vi "Halvorsen_Effect_Graph.vi"() -> ()   [LabVIEW 2016]
panel:
  in  "Parameters array":dbl[](array[numeric])=[1.4, 1.4, 1.4]
  in  "last_point_Thomas":dbl[](array[numeric])=[2.3727475682665875, 0.23609824454436878, 0.4447912442126299]
  out "Efficiency plot":cluster{dbl[], dbl[]}[](graph)=[{[0.003543503530615683, 0.008857469273654535, 0.00019032089210001206, 1.3154265970568985e-05, 7.569954419870983e-07, 2.611584956422264e-08, 5.111791074846327e-10, 1.2810097409899129e-09, 1.4983661356938417e-09, 8.704238501746543e-11], [0.0006568757962668315, 0.0006969041642150842, 0.001332226223894395, 0.0013178570661693811, 0.001516972541139694, 0.0019039134404010838, 0.002382201128966699, 0.0033203018756466918, 0.004479071834794013, 0.006073022008422413]}, {[0.05292939277385792, 0.005366821516305654, 0.00032764804221647705, 2.8472873719995087e-05, 1.7555059222208518e-06, 2.2173371174251578e-07, 4.046899467880833e-09, 2.1493117845000048e-09, 1.62941200420686e-09, 7.302730760301067e-09], [0.0007903036921561579, 0.0010448430630276562, 0.001373280961161072, 0.0016955606479314156, 0.003905331881469465, 0.0027578519757298636, 0.004559128571600013, 0.00517905510514538, 0.007503779601393035, 0.010119992733962135]}, {[0.002038488022454064, 0.000645465458210278, 0.00017338121373700052, 3.264021324537677e-05, 2.183623841080202e-06, 1.9365539284403195e-07, 2.508911679074605e-08, 3.0422395440576762e-09, 1.1221599069650436e-10, 1.6048322905065433e-09], [0.0009863400628091767, 0.0013722545927521423, 0.0017335362808807986, 0.0021943757055851165, 0.0030134177141007967, 0.0041157374098474975, 0.005651184582347923, 0.007658761235688871, 0.010887716319302854, 0.015299047837288526]}, {[0.0065546151240054125, 0.003030290222989306, 0.0008963869972767443, 8.930764045777448e-05, 2.652903337131928e-05, 1.0284405279190207e-06, 9.203396690137426e-08, 1.058326598406588e-08, 1.8330857120193038e-09, 8.540691445443122e-11], [0.0007246161130751716, 0.0009391271141794277, 0.0012429321695890394, 0.0016863233322510496, 0.0021256090221868362, 0.0027855639227709617, 0.0037452184060384752, 0.004844458995648893, 0.006607759961298143, 0.00915212730251369]}, {[0.031777470957385985, 0.0021554762412673728, 9.17895270926683e-05, 1.7052624686084191e-06, 6.452919290133345e-07, 4.7099078030656e-08, 8.99697945269555e-09, 4.212593948523254e-10, 1.4960189944277468e-10, 8.913127927436747e-10], [0.000523447900377505, 0.0006219792694537318, 0.0008467539555567782, 0.0011053988009734894, 0.0014461531200140598, 0.001842331334046321, 0.002354489181925601, 0.0033921476651812554, 0.0042563498855088255, 0.00598783342866227]}, {[0.01953779155905403, 0.011210076118577949, 0.0003345025752221787, 1.698158066222403e-06, 1.2746234512715955e-06, 2.029307378175867e-08, 3.577829362814558e-10, 3.945270287029524e-10, 2.68884023315538e-10, 2.253025074843069e-09], [0.000610689216046012, 0.0007636181126144947, 0.0014882342256896663, 0.0017171143863379257, 0.0023165135498857126, 0.0021687164962713723, 0.0025628419725762797, 0.0038991736710158875, 0.005071286419479293, 0.006304981274297461]}, {[0.644522862841223, 0.07384111446896484, 0.038699076952541156, 0.00422549784591777, 0.0006539084545961815, 0.0001447132168707633, 3.4362296547381575e-05, 6.549119527339312e-06, 6.89087435666376e-06, 1.0243970291599666e-05], [0.0008467539555567782, 0.0011567172214199672, 0.0017591954920135322, 0.0029518356086555286, 0.004991229681763798, 0.008791871982793964, 0.015572061841339746, 0.0268436399546772, 0.045662105143492226, 0.06235393494262098]}, {[0.06903372684326185, 0.00020304900818616015, 8.637150762520324e-05, 1.689029168945209e-06, 8.057455570285068e-07, 2.9659954301410987e-08, 2.4135215284240776e-09, 1.1473823618093083e-09, 6.606131463009407e-10, 6.428058997780049e-10], [0.0005727135840061237, 0.0006989569010329433, 0.0009688917998573743, 0.0012860396445830702, 0.0016996661224766285, 0.003623080562647374, 0.002643925078700704, 0.00331311729587469, 0.0048054569961095694, 0.006534887802445155]}, {[0.009934991568151866, 0.001930410234965607, 5.014437765295048e-05, 1.7981970136881245e-05, 5.418162911083816e-06, 1.00173853871348e-06, 2.4670319318787825e-07, 3.898500256142404e-08, 5.109251324047994e-09, 3.051511094268924e-10], [0.005962174217529537, 0.008118574292893754, 0.009580122939041757, 0.012024932541862654, 0.01608421968830953, 0.021048763790531666, 0.02561712967872154, 0.03248045537930011, 0.04417387091780256, 0.06094370471782895]}]
  in  "Multipliers":i32[](array[numeric])=[2, 2, 2, 2, 2, 2, 2, 2, 2, 2, 2, 2, 2]
  in  "Methods":u16[](array[ring])=[0, 4, 5, 9, 1, 2, 6, 3, 10] items=["ECD1", "ECD2", "ECD3", "ECD4", "EMP", "LIMP", "SEMP", "SIMP", "Euler", "MEMP", "IMP", "IEuler", "MSEMP"]
  in  "Tab Control":enum32{"Variable step", "Fixed Step"}(tab)
  in  "Tolerances":dbl[](array[numeric])=[0.0001, 1e-05, 1e-06, 1e-07, 1e-08, 1e-09, 1e-10, 1e-11, 1e-12, 1e-13]
  in  "Max Steps":dbl[](array[numeric])=[2.0, 2.0, 2.0, 2.0, 2.0, 2.0, 2.0, 2.0, 2.0, 2.0]
  in  "Start steps":dbl[](array[numeric])=[0.01, 0.01, 0.01, 0.01, 0.01, 0.01, 0.01, 0.01, 0.01, 0.04]
  in  "Min Steps":dbl[](array[numeric])=[0.001, 0.001, 0.001, 0.001, 0.001, 0.001, 0.001, 0.001, 0.001, 0.001]
  in  "Tolerances 2":dbl[](array[numeric])=[1e-06, 1e-06, 1e-06, 1e-06, 1e-06, 1e-06, 1e-06, 1e-06, 1e-06]
  in  "Start steps 2":dbl[](array[numeric])=[2.0, 1.0, 0.4, 0.3, 0.2, 0.1, 0.08, 0.05, 0.02, 0.01]
  out "Rejected":i32[][](array[numeric])=[[11, 16, 10, 11, 8, 11, 14, 10, 11], [12, 18, 13, 14, 9, 9, 15, 12, 12], [14, 24, 13, 18, 13, 16, 14, 16, 15], [16, 19, 17, 22, 16, 16, 17, 19, 16], [16, 14, 19, 18, 16, 17, 18, 17, 21], [15, 6, 16, 12, 14, 18, 19, 19, 25], [7, 3, 9, 8, 8, 12, 20, 11, 17], [5, 2, 1, 2, 2, 5, 22, 6, 2], [5, 2, 1, 0, 0, 3, 24, 4, 2], [5, 2, 2, 1, 1, 3, 21, 3, 1]]
  in  "Points count":i32=1
  in  "Ext.Type":u16(ring) items=["FNode", "MathScript", "ECD8 Arrays", "ECD8 Fnode", "ECD8 FnodeDiv", "FNode Exp"]
  in  "?":bool
  in  "n_2":i32[](array[numeric])=[2, 3, 4, 5, 8, 10, 12, 14, 16, 10, 11]
  in  "n_1":i32[](array[numeric])=[1, 2, 3, 4, 5, 6, 7, 8, 9, 10, 11]
  out "Times":dbl[][](array[numeric])=[[0.0006568757962668315, 0.0007903036921561579, 0.0009863400628091767, 0.0007246161130751716, 0.000523447900377505, 0.000610689216046012, 0.0008467539555567782, 0.0005727135840061237, 0.005962174217529537], [0.0006969041642150842, 0.0010448430630276562, 0.0013722545927521423, 0.0009391271141794277, 0.0006219792694537318, 0.0007636181126144947, 0.0011567172214199672, 0.0006989569010329433, 0.008118574292893754], [0.001332226223894395, 0.001373280961161072, 0.0017335362808807986, 0.0012429321695890394, 0.0008467539555567782, 0.0014882342256896663, 0.0017591954920135322, 0.0009688917998573743, 0.009580122939041757], [0.0013178570661693811, 0.0016955606479314156, 0.0021943757055851165, 0.0016863233322510496, 0.0011053988009734894, 0.0017171143863379257, 0.0029518356086555286, 0.0012860396445830702, 0.012024932541862654], [0.001516972541139694, 0.003905331881469465, 0.0030134177141007967, 0.0021256090221868362, 0.0014461531200140598, 0.0023165135498857126, 0.004991229681763798, 0.0016996661224766285, 0.01608421968830953], [0.0019039134404010838, 0.0027578519757298636, 0.0041157374098474975, 0.0027855639227709617, 0.001842331334046321, 0.0021687164962713723, 0.008791871982793964, 0.003623080562647374, 0.021048763790531666], [0.002382201128966699, 0.004559128571600013, 0.005651184582347923, 0.0037452184060384752, 0.002354489181925601, 0.0025628419725762797, 0.015572061841339746, 0.002643925078700704, 0.02561712967872154], [0.0033203018756466918, 0.00517905510514538, 0.007658761235688871, 0.004844458995648893, 0.0033921476651812554, 0.0038991736710158875, 0.0268436399546772, 0.00331311729587469, 0.03248045537930011], [0.004479071834794013, 0.007503779601393035, 0.010887716319302854, 0.006607759961298143, 0.0042563498855088255, 0.005071286419479293, 0.045662105143492226, 0.0048054569961095694, 0.04417387091780256], [0.006073022008422413, 0.010119992733962135, 0.015299047837288526, 0.00915212730251369, 0.00598783342866227, 0.006304981274297461, 0.06235393494262098, 0.006534887802445155, 0.06094370471782895]] format="%#_10f"
  out "Steps":i32[][](array[numeric])=[[28, 50, 28, 43, 27, 27, 55, 27, 27], [34, 66, 37, 58, 34, 33, 79, 34, 35], [45, 91, 49, 77, 46, 45, 130, 46, 45], [61, 120, 65, 104, 62, 61, 225, 66, 59], [83, 164, 89, 140, 84, 83, 396, 86, 80], [115, 225, 121, 191, 114, 116, 702, 117, 108], [156, 311, 166, 263, 156, 156, 1249, 159, 146], [216, 431, 229, 364, 215, 215, 2200, 220, 200], [299, 599, 320, 505, 298, 298, 3548, 305, 278], [415, 831, 444, 701, 414, 413, 4777, 424, 386]]
  out "Errors":dbl[][](array[numeric])=[[0.003543503530615683, 0.05292939277385792, 0.002038488022454064, 0.0065546151240054125, 0.031777470957385985, 0.01953779155905403, 0.644522862841223, 0.06903372684326185, 0.009934991568151866], [0.008857469273654535, 0.005366821516305654, 0.000645465458210278, 0.003030290222989306, 0.0021554762412673728, 0.011210076118577949, 0.07384111446896484, 0.00020304900818616015, 0.001930410234965607], [0.00019032089210001206, 0.00032764804221647705, 0.00017338121373700052, 0.0008963869972767443, 9.17895270926683e-05, 0.0003345025752221787, 0.038699076952541156, 8.637150762520324e-05, 5.014437765295048e-05], [1.3154265970568985e-05, 2.8472873719995087e-05, 3.264021324537677e-05, 8.930764045777448e-05, 1.7052624686084191e-06, 1.698158066222403e-06, 0.00422549784591777, 1.689029168945209e-06, 1.7981970136881245e-05], [7.569954419870983e-07, 1.7555059222208518e-06, 2.183623841080202e-06, 2.652903337131928e-05, 6.452919290133345e-07, 1.2746234512715955e-06, 0.0006539084545961815, 8.057455570285068e-07, 5.418162911083816e-06], [2.611584956422264e-08, 2.2173371174251578e-07, 1.9365539284403195e-07, 1.0284405279190207e-06, 4.7099078030656e-08, 2.029307378175867e-08, 0.0001447132168707633, 2.9659954301410987e-08, 1.00173853871348e-06], [5.111791074846327e-10, 4.046899467880833e-09, 2.508911679074605e-08, 9.203396690137426e-08, 8.99697945269555e-09, 3.577829362814558e-10, 3.4362296547381575e-05, 2.4135215284240776e-09, 2.4670319318787825e-07], [1.2810097409899129e-09, 2.1493117845000048e-09, 3.0422395440576762e-09, 1.058326598406588e-08, 4.212593948523254e-10, 3.945270287029524e-10, 6.549119527339312e-06, 1.1473823618093083e-09, 3.898500256142404e-08], [1.4983661356938417e-09, 1.62941200420686e-09, 1.1221599069650436e-10, 1.8330857120193038e-09, 1.4960189944277468e-10, 2.68884023315538e-10, 6.89087435666376e-06, 6.606131463009407e-10, 5.109251324047994e-09], [8.704238501746543e-11, 7.302730760301067e-09, 1.6048322905065433e-09, 8.540691445443122e-11, 8.913127927436747e-10, 2.253025074843069e-09, 1.0243970291599666e-05, 6.428058997780049e-10, 3.051511094268924e-10]] format="%#_9e"
  in  "Время, с":dbl=5.0
  in  "k":i32=4
  in  "Error Analysis":u16(ring)=2 items=["Max", "Max_Norm", "Norm", "Last Value", "Last Constant"]
  # "0 ECD1\n1 ECD2\n2 ECD3\n3 ECD4\n4 EMP\n5 LIMP\n6 SEMP\n7 SIMP\n8 Euler\n9 Euler-Cromer\n10 MECD1\n11 MECD2\n12 MECD3\n13 MECD4\n14 MEMP\n15 MLIMP\n16 MSEMP\n17 MSIMP"
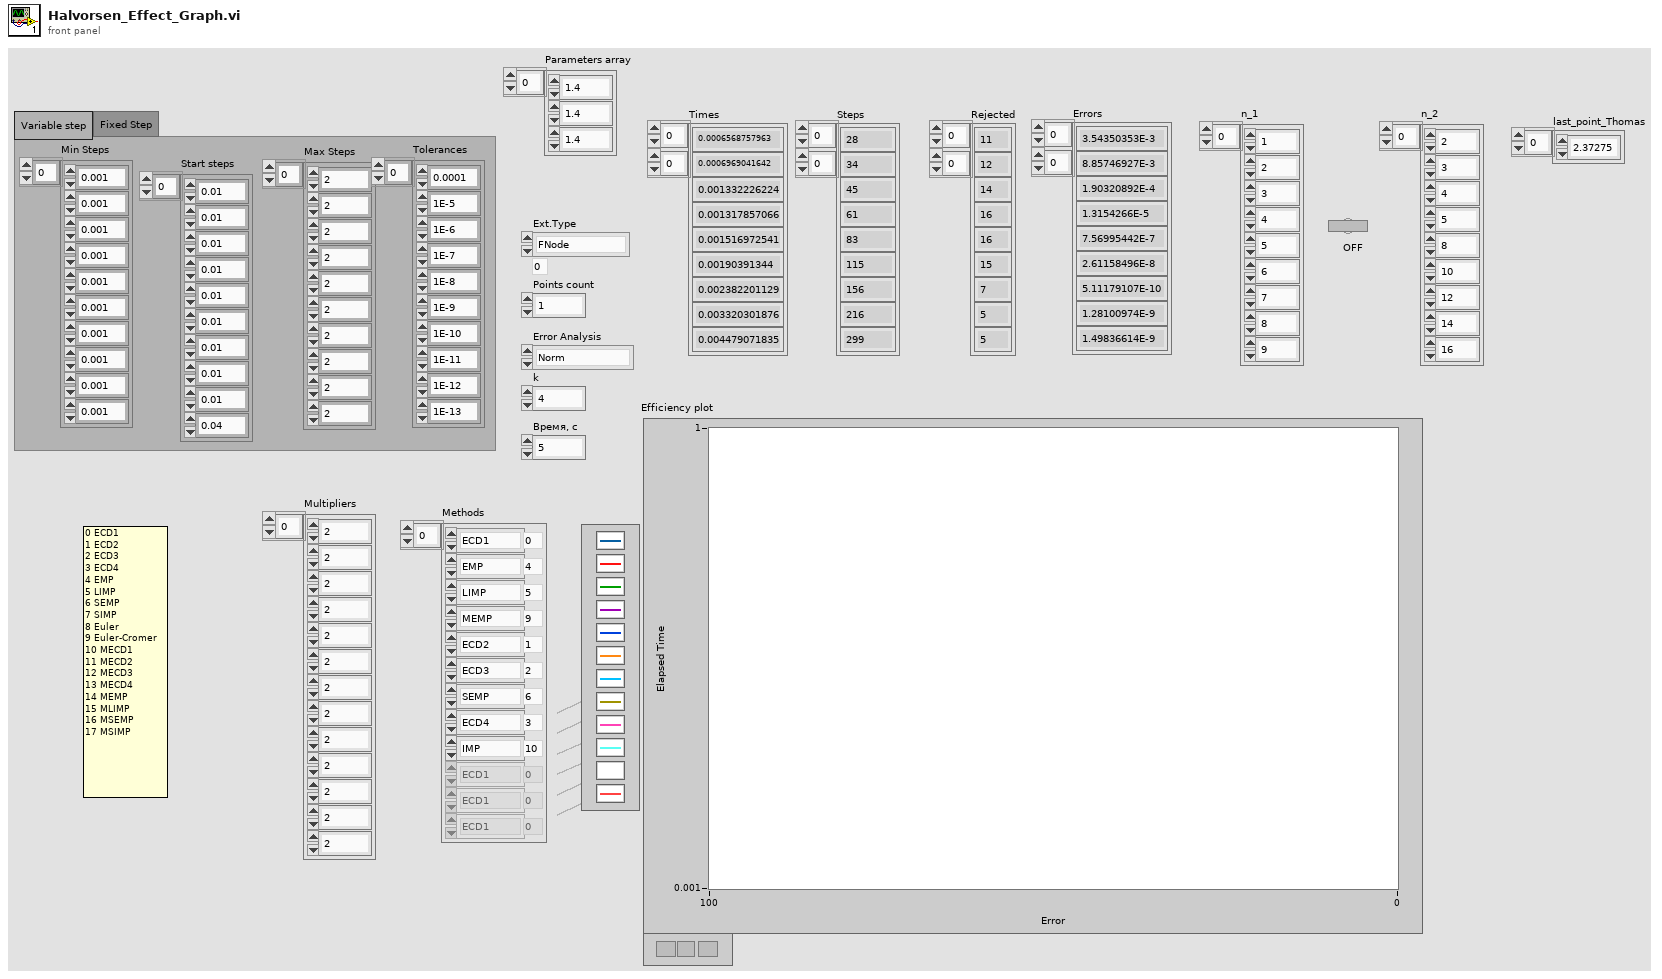
[diagram p1: front panel]
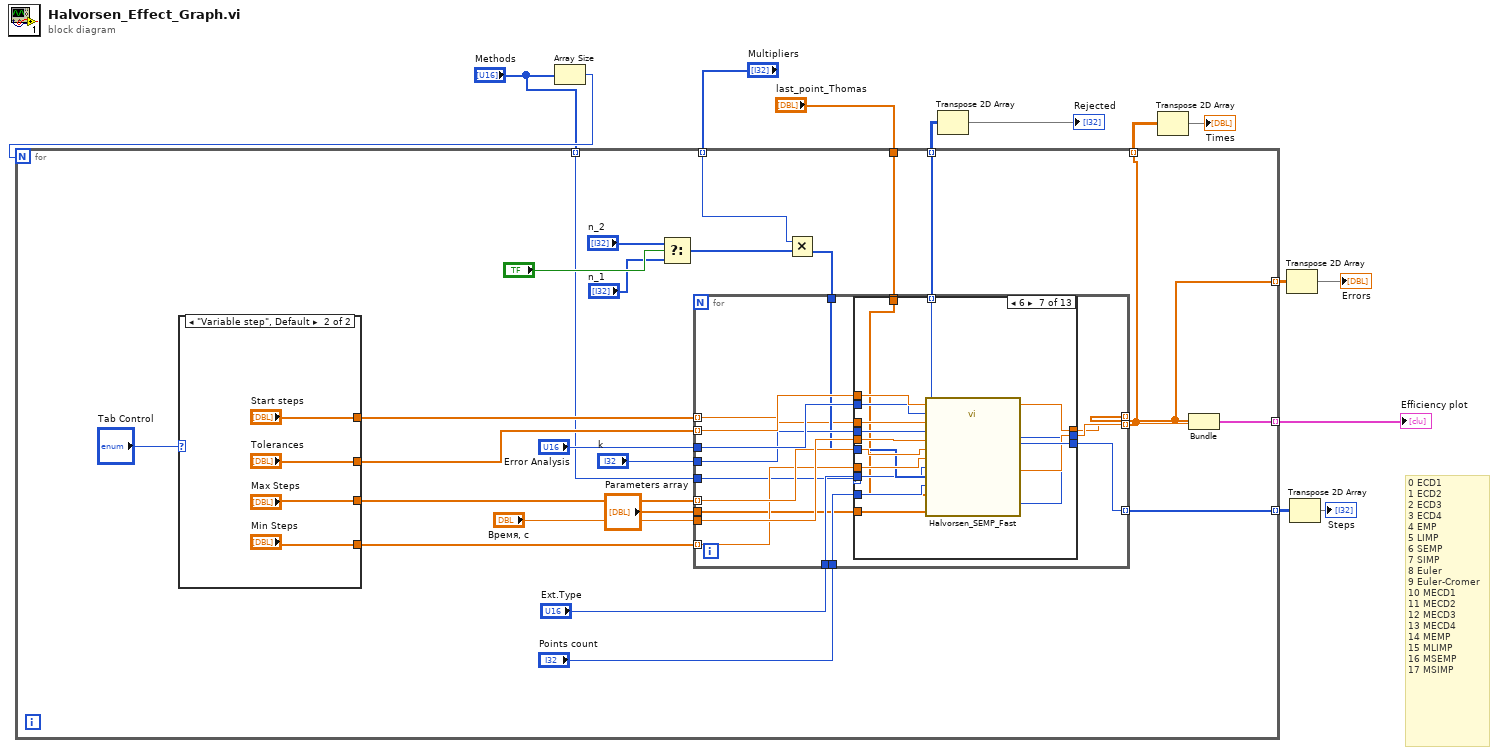
[diagram p0: block diagram]
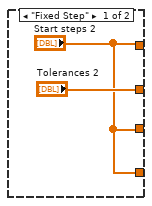
[diagram p2: hidden frame]
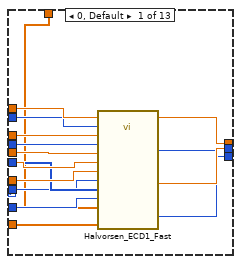
[diagram p3: hidden frame]
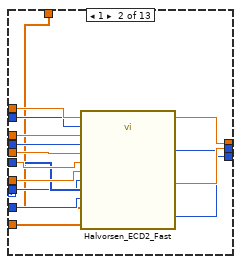
[diagram p4: hidden frame]
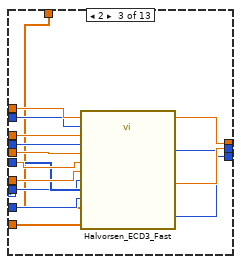
[diagram p5: hidden frame]
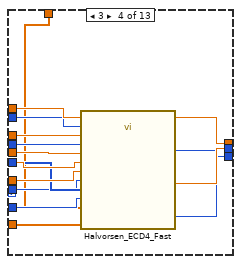
[diagram p6: hidden frame]
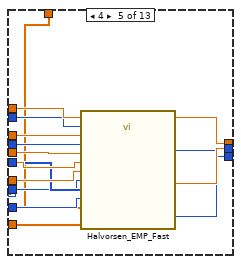
[diagram p7: hidden frame]
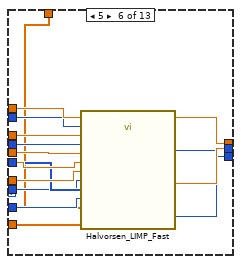
[diagram p8: hidden frame]
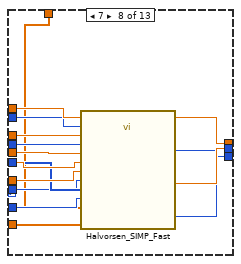
[diagram p9: hidden frame]
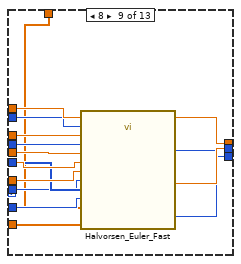
[diagram p10: hidden frame]
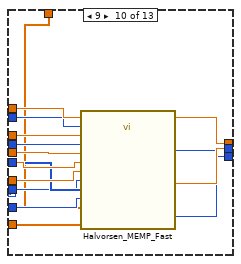
[diagram p11: hidden frame]
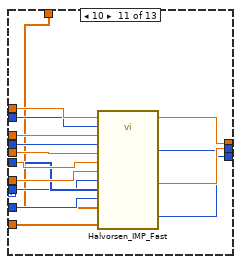
[diagram p12: hidden frame]
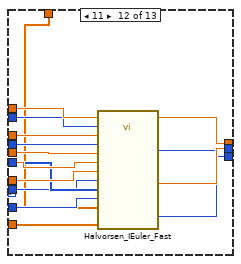
[diagram p13: hidden frame]
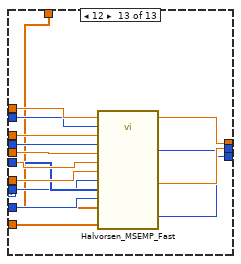
[diagram p14: hidden frame]
diagram:
  # "0 ECD1\n1 ECD2\n2 ECD3\n3 ECD4\n4 EMP\n5 LIMP\n6 SEMP\n7 SIMP\n8 Euler\n9 Euler-Cromer\n10 MECD1\n11 MECD2\n12 MECD3\n13 MECD4\n14 MEMP\n15 MLIMP\n16 MSEMP\n17 MSIMP"
  n1 = Array Size(array="Methods") -> (size(s)=w5:i32)
  n2 = for {
    N: w5 -> [_]
    tunnel: [w22] -> w2 mode=indexing
    tunnel: [w21] -> w13 mode=indexing
    tunnel: [w20] -> w12 mode=indexing
    tunnel: [w19] -> w11 mode=indexing
    tunnel: [w18] -> w10 mode=indexing
    tunnel: "Methods" -> [w17] mode=indexing
    tunnel: "Multipliers" -> [w16] mode=indexing
    tunnel: "last_point_Thomas" -> [w15]
    n3 = case shown="\"Variable step\", Default" "Tab Control" {
      tunnel: ["Tolerances 2" "Tolerances"] -> w37
      tunnel: ["Start steps 2" "Start steps"] -> w26
      tunnel: ["Start steps 2" "Max Steps"] -> w25
      tunnel: ["Start steps 2" "Min Steps"] -> w24
      frame "Fixed Step" {
      }
      frame "Variable step", Default {
      }
    }
    n4 = Select(t="n_2", s="?", f="n_1") -> (s? t:f=w32:i32[])
    n5 = Multiply(x=w16, y=w32) -> (x*y=w33:i32[])
    n6 = for {
      tunnel: w37 -> [w60] mode=indexing
      tunnel: "Error Analysis" -> [w59]
      tunnel: "k" -> [w58]
      tunnel: "Время, с" -> [w57]
      tunnel: w25 -> [w56] mode=indexing
      tunnel: w24 -> [w55] mode=indexing
      tunnel: w33 -> [w54]
      tunnel: [w53] -> w18 mode=indexing
      tunnel: [w52] -> w19 mode=indexing
      tunnel: [w51] -> w21 mode=indexing
      tunnel: "Ext.Type" -> [w50]
      tunnel: "Points count" -> [w49]
      tunnel: [w48] -> w20 mode=indexing
      tunnel: w26 -> [w47] mode=indexing
      tunnel: w17 -> [w46]
      tunnel: w15 -> [w45]
      tunnel: "Parameters array" -> [w44]
      n7 = case shown="6" w46 {
        tunnel: w60 -> [w76 w92 w108 w124 w140 w156 w172 w188 w204 w220 w236 w252 w268]
        tunnel: w59 -> [w75 w91 w107 w123 w139 w155 w171 w187 w203 w219 w235 w251 w267]
        tunnel: w58 -> [w74 w90 w106 w122 w138 w154 w170 w186 w202 w218 w234 w250 w266]
        tunnel: w57 -> [w73 w89 w105 w121 w137 w153 w169 w185 w201 w217 w233 w249 w265]
        tunnel: w56 -> [w72 w88 w104 w120 w136 w152 w168 w184 w200 w216 w232 w248 w264]
        tunnel: w55 -> [w71 w87 w103 w119 w135 w151 w167 w183 w199 w215 w231 w247 w263]
        tunnel: w54 -> [w70 w86 w102 w118 w134 w150 w166 w182 w198 w214 w230 w246 w262]
        tunnel: [w69 w85 w101 w117 w133 w149 w165 w181 w197 w213 w229 w245 w261] -> w53
        tunnel: [w68 w84 w100 w116 w132 w148 w164 w180 w196 w212 w228 w244 w260] -> w52
        tunnel: [w67 w83 w99 w115 w131 w147 w163 w179 w195 w211 w227 w243 w259] -> w51
        tunnel: w50 -> [w66 w82 w98 w114 w130 w146 w162 w178 w194 w210 w226 w242 w258]
        tunnel: w49 -> [w65 w81 w97 w113 w129 w145 w161 w177 w193 w209 w225 w241 w257]
        tunnel: [w64 w80 w96 w112 w128 w144 w160 w176 w192 w208 w224 w240 w256] -> w48
        tunnel: w47 -> [w63 w79 w95 w111 w127 w143 w159 w175 w191 w207 w223 w239 w255]
        tunnel: w45 -> [w62 w78 w94 w110 w126 w142 w158 w174 w190 w206 w222 w238 w254]
        tunnel: w44 -> [w61 w77 w93 w109 w125 w141 w157 w173 w189 w205 w221 w237 w253]
        frame 0, Default {
          n8 = call "Halvorsen_ECD1_Fast.vi"("tolerance"=w76, "Error Analysis"=w75, "Шаг h, с"=w63, "k"=w74, "Время, с"=w73, "Hmax"=w72, "b"=w61, "last_point_Thomas"=w62, "Hmin"=w71, "Points count"=w65, "n"=w70, "Ext.Type"=w66) -> ("Elapsed Time"=w69:dbl, "Number of steps"=w67:i32, "Error Estimation"=w68:dbl, "Rejected steps"=w64:i32)  [unwired: 4 in]
        }
        frame 1 {
          n9 = call "Halvorsen_ECD2_Fast.vi"("tolerance"=w92, "Error Analysis"=w91, "Шаг h, с"=w79, "k"=w90, "Время, с"=w89, "Hmax"=w88, "b"=w77, "last_point_Thomas"=w78, "Hmin"=w87, "Points count"=w81, "n"=w86, "Ext.Type"=w82) -> ("Elapsed Time"=w85:dbl, "Number of steps"=w83:i32, "Error Estimation"=w84:dbl, "Rejected steps"=w80:i32)  [unwired: 4 in]
        }
        frame 2 {
          n10 = call "Halvorsen_ECD3_Fast.vi"("tolerance"=w108, "Error Analysis"=w107, "Шаг h, с"=w95, "k"=w106, "Время, с"=w105, "Hmax"=w104, "b"=w93, "last_point_Thomas"=w94, "Hmin"=w103, "Points count"=w97, "n"=w102, "Ext.Type"=w98) -> ("Elapsed Time"=w101:dbl, "Number of steps"=w99:i32, "Error Estimation"=w100:dbl, "Rejected steps"=w96:i32)  [unwired: 4 in]
        }
        frame 3 {
          n11 = call "Halvorsen_ECD4_Fast.vi"("tolerance"=w124, "Error Analysis"=w123, "Шаг h, с"=w111, "k"=w122, "Время, с"=w121, "Hmax"=w120, "b"=w109, "last_point_Thomas"=w110, "Hmin"=w119, "Points count"=w113, "n"=w118, "Ext.Type"=w114) -> ("Elapsed Time"=w117:dbl, "Number of steps"=w115:i32, "Error Estimation"=w116:dbl, "Rejected steps"=w112:i32)  [unwired: 4 in]
        }
        frame 4 {
          n12 = call "Halvorsen_EMP_Fast.vi"("tolerance"=w140, "Error Analysis"=w139, "Шаг h, с"=w127, "k"=w138, "Время, с"=w137, "Hmax"=w136, "Parameter"=w125, "last_point_Thomas"=w126, "Hmin"=w135, "Points count"=w129, "n"=w134, "Ext.Type"=w130) -> ("Elapsed Time"=w133:dbl, "Number of steps"=w131:i32, "Error Estimation"=w132:dbl, "Rejected steps"=w128:i32)  [unwired: 4 in]
        }
        frame 5 {
          n13 = call "Halvorsen_LIMP_Fast.vi"("tolerance"=w156, "Error Analysis"=w155, "Шаг h, с"=w143, "k"=w154, "Время, с"=w153, "Hmax"=w152, "Parameter"=w141, "last_point_Thomas"=w142, "Hmin"=w151, "Points count"=w145, "n"=w150, "Ext.Type"=w146) -> ("Elapsed Time"=w149:dbl, "Number of steps"=w147:i32, "Error Estimation"=w148:dbl, "Rejected steps"=w144:i32)  [unwired: 4 in]
        }
        frame 6 {
          n14 = call "Halvorsen_SEMP_Fast.vi"("tolerance"=w172, "Error Analysis"=w171, "Шаг h, с"=w159, "k"=w170, "Время, с"=w169, "Hmax"=w168, "Parameter"=w157, "last_point_Thomas"=w158, "Hmin"=w167, "Points count"=w161, "n"=w166, "Ext.Type"=w162) -> ("Elapsed Time"=w165:dbl, "Number of steps"=w163:i32, "Error Estimation"=w164:dbl, "Rejected steps"=w160:i32)  [unwired: 4 in]
        }
        frame 7 {
          n15 = call "Halvorsen_SIMP_Fast.vi"("tolerance"=w188, "Error Analysis"=w187, "Шаг h, с"=w175, "k"=w186, "Время, с"=w185, "Hmax"=w184, "Parameters"=w173, "last_point_Thomas"=w174, "Hmin"=w183, "Points count"=w177, "n"=w182, "Ext.Type"=w178) -> ("Elapsed Time"=w181:dbl, "Number of steps"=w179:i32, "Error Estimation"=w180:dbl, "Rejected steps"=w176:i32)  [unwired: 4 in]
        }
        frame 8 {
          n16 = call "Halvorsen_Euler_Fast.vi"("tolerance"=w204, "Error Analysis"=w203, "Шаг h, с"=w191, "k"=w202, "Время, с"=w201, "Hmax"=w200, "Parameters"=w189, "last_point_Thomas"=w190, "Hmin"=w199, "Points count"=w193, "n"=w198, "Ext.Type"=w194) -> ("Elapsed Time"=w197:dbl, "Number of steps"=w195:i32, "Error Estimation"=w196:dbl, "Rejected steps"=w192:i32)  [unwired: 4 in]
        }
        frame 9 {
          n17 = call "Halvorsen_MEMP_Fast.vi"("tolerance"=w220, "Error Analysis"=w219, "Шаг h, с"=w207, "k"=w218, "Время, с"=w217, "Hmax"=w216, "Parameter"=w205, "last_point_Thomas"=w206, "Hmin"=w215, "Points count"=w209, "n"=w214, "Ext.Type"=w210) -> ("Elapsed Time"=w213:dbl, "Number of steps"=w211:i32, "Error Estimation"=w212:dbl, "Rejected steps"=w208:i32)  [unwired: 4 in]
        }
        frame 10 {
          n18 = call "Halvorsen_IMP_Fast.vi"("tolerance"=w236, "Error Analysis"=w235, "Шаг h, с"=w223, "k"=w234, "Время, с"=w233, "Hmax"=w232, "Parameter"=w221, "last_point_Thomas"=w222, "Hmin"=w231, "Points count"=w225, "n"=w230, "Ext.Type"=w226) -> ("Elapsed Time"=w229:dbl, "Number of steps"=w227:i32, "Error Estimation"=w228:dbl, "Rejected steps"=w224:i32)  [unwired: 4 in]
        }
        frame 11 {
          n19 = call "Halvorsen_IEuler_Fast.vi"("tolerance"=w252, "Error Analysis"=w251, "Шаг h, с"=w239, "k"=w250, "Время, с"=w249, "Hmax"=w248, "Parameters"=w237, "last_point_Thomas"=w238, "Hmin"=w247, "Points count"=w241, "n"=w246, "Ext.Type"=w242) -> ("Elapsed Time"=w245:dbl, "Number of steps"=w243:i32, "Error Estimation"=w244:dbl, "Rejected steps"=w240:i32)  [unwired: 4 in]
        }
        frame 12 {
          n20 = call "Halvorsen_MSEMP_Fast.vi"("tolerance"=w268, "Error Analysis"=w267, "Шаг h, с"=w255, "k"=w266, "Время, с"=w265, "Hmax"=w264, "Parameter"=w253, "last_point_Thomas"=w254, "Hmin"=w263, "Points count"=w257, "n"=w262, "Ext.Type"=w258) -> ("Elapsed Time"=w261:dbl, "Number of steps"=w259:i32, "Error Estimation"=w260:dbl, "Rejected steps"=w256:i32)  [unwired: 4 in]
        }
      }
    }
    n21 = Bundle(w19, w18) -> (w22:cluster{dbl[], dbl[]})  [unwired: 1 in]
  }
  "Efficiency plot" <- w2
  n22 = Transpose 2D Array(2D array=w12) -> (transposed array=→"Rejected":i32[][])
  n23 = Transpose 2D Array(2D array=w10) -> (transposed array=→"Times":dbl[][])
  n24 = Transpose 2D Array(2D array=w11) -> (transposed array=→"Errors":dbl[][])
  n25 = Transpose 2D Array(2D array=w13) -> (transposed array=→"Steps":i32[][])
